vi "SCCAPI Get Advanced Command Options.vi"(7 "advanced options in":variant, 8 "error in (no error)":errorcluster, 10 "command":T1 items=["GET", "CHECKOUT", "CHECKIN", "UNDOCHECKOUT", "ADD", "REMOVE", "COMPARE", "FILEHISTORY", "FILEPROPERTIES", "CONFIGOPTIONS"], 11 "source control reference in":T2) -> (0 "error out":errorcluster, 1 "dialog box cancelled?":bool, 2 "status message":string, 3 "source control reference out":T2, 5 "advanced options out":variant)   [LabVIEW 2017, in "NI_SCC.lvlib"]
uses:
  <vilib>/SourceControl/sccapi/NI_SCC.lvlib
  <vilib>/SourceControl/sccapi/SCCAPI Refnum.ctl
  <vilib>/SourceControl/sccapi/SCCAPI Command.ctl
  <vilib>/SourceControl/sccapi/SCCAPI SCC Operations.ctl
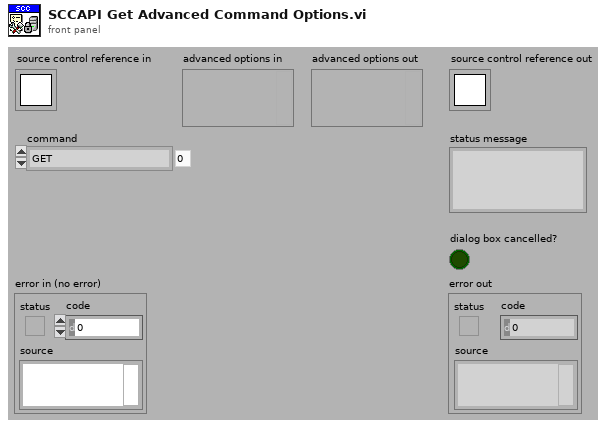
[diagram p1: front panel]
types:
  T1 = typedef "NI_SCC.lvlib/SCCAPI Command.ctl" = i32
  T2 = typedef "NI_SCC.lvlib/SCCAPI Refnum.ctl" = refnum<k1>
  T3 = typedef "NI_SCC.lvlib/SCCAPI SCC Operations.ctl" = enum16{"Add", "Check In", "Check Out", "Close Project", "Compare Files", "Compare VIs", "Configure Project", "File History", "File Properties", "File Status", "Find All Providers", "Get Advanced Command Options", "Get File Copy", "Get Latest Version", "Get Project Name", "Get StaticVI Path", "Initialize", "Not A Source Control Reference", "Open Project", "Provider Supports Functionality", "Remove", "Run Provider", "Undo Check Out", "Uninitialize", "Is File In Local Path"}
  T4 = typedef "SCCAPI Refnum.ctl" = refnum<k1>
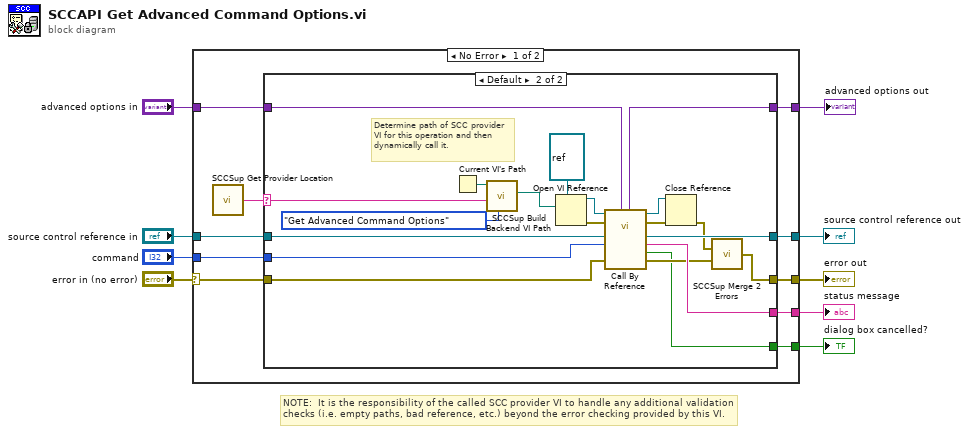
[diagram p0: block diagram]
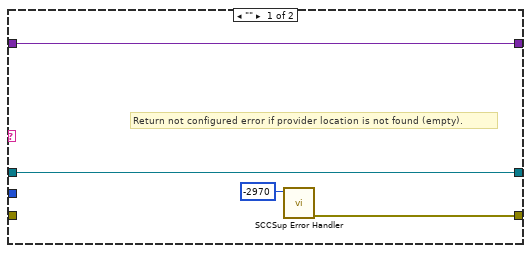
[diagram p2: hidden frame]
diagram:
  # "NOTE:  It is the responsibility of the called SCC provider VI to handle any additional validation checks (i.e. empty paths, bad reference, etc.) beyond the error checking provided by this VI."
  n1 = case shown="No Error" "error in (no error)" {
    selector: "error in (no error)" -> [w13 w46]
    tunnel: [w19 w46] -> w8
    tunnel: "source control reference in" -> [w18 w45]
    tunnel: [w17 _] -> w6
    tunnel: [w16 w45] -> w5
    tunnel: "command" -> [w15 _]
    tunnel: [w12 _] -> w3
    tunnel: [w11 w44] -> w2
    tunnel: "advanced options in" -> [w10 w44]
    frame No Error {
      n2 = call <vilib>:"SCCSup Get Provider Location.vi"() -> ("provider location"=w14:string)  [unwired: 6 in]
      n3 = case shown="Default" w14 {
        selector: w14 -> [_ w28]
        tunnel: [w21 w43] -> w19
        tunnel: w18 -> [w23 w35]
        tunnel: [_ w42] -> w17
        tunnel: [w23 w36] -> w16
        tunnel: w15 -> [_ w34]
        tunnel: w13 -> [_ w27]
        tunnel: [_ w26] -> w12
        tunnel: [w20 w25] -> w11
        tunnel: w10 -> [w20 w24]
        frame "" {
          # "Return not configured error if provider location is not found (empty)."
          n4 = call <vilib>:"SCCSup Error Handler.vi"("scc error code"=-2970 ("code")) -> ("error out"=w21:errorcluster)  [unwired: 10 in]
        }
        frame Default {
          # "Determine path of SCC provider VI for this operation and then dynamically call it."
          n5 = Current VI's Path() -> (path=w29:path)
          n6 = call <vilib>:"SCCSup Build Backend VI Path.vi"("scc operation"=SCCAPI_SCC_Operations."Get Advanced Command Options", "provider location"=w28, "caller path"=w29) -> ("scc backend VI path"=w31:path)  [unwired: 8 in]
          n7 = Open VI Reference(type specifier VI Refnum (for type only)=refnum<vi> refnum, vi path=w31) -> (vi reference=w40:refnum<vi>, error out=w39:errorcluster)  [unwired: 4 in]
          n8 = call-by-ref "?"(reference=w40, error in=w39, "advanced options in"=w24, "error in (no error)"=w27, "command"=w34, "source control reference in"=w35) -> (reference out=w38:refnum<vi>, error out=w37:errorcluster, 0:"error out"=w32:errorcluster, "dialog box cancelled?"=w26:bool, "status message"=w42:string, "source control reference out"=w36:T4, "advanced options"=w25:variant)  [unwired: 3 in]
          n9 = Close Reference(reference=w38, error in (no error)=w37) -> (error out=w33:errorcluster)
          n10 = call <vilib>:"SCCSup Merge 2 Errors.vi"("Error IO 1"=w33, "Error IO 2"=w32) -> ("Error IO out"=w43:errorcluster)  [unwired: 13 in]
        }
      }
    }
    frame Error {
    }
  }
  "error out" <- w8
  "status message" <- w6
  "source control reference out" <- w5
  "dialog box cancelled?" <- w3
  "advanced options out" <- w2
